vi "logTof.vi"(8 "ToF Reading":T1, 9 "Index":i32) -> ()   [LabVIEW 2014]
uses:
  Type Defs/tofReading.ctl
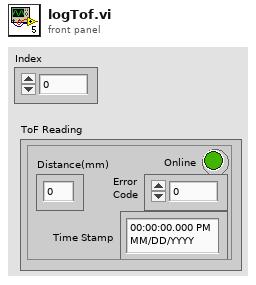
[diagram p1: front panel]
types:
  T1 = typedef "tofReading.ctl" = cluster{"Distance(mm)":u8, "Online":bool, "Error\nCode":u8, "Time Stamp":timestamp}
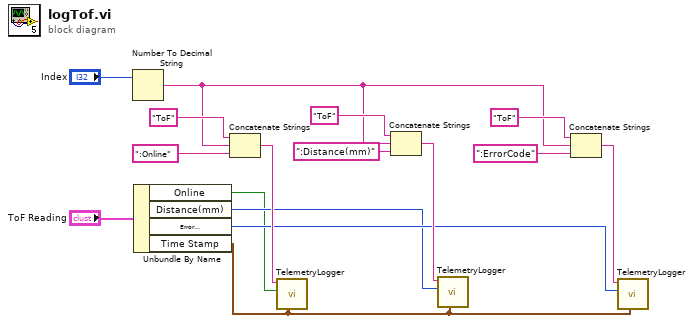
[diagram p0: block diagram]
diagram:
  n1 = Number To Decimal String(number="Index") -> (decimal integer string=w6:string)  [unwired: 1 in]
  n2 = Unbundle By Name("ToF Reading") -> ("Online"=w1:bool, "Distance(mm)"=w2:u8, "Error\nCode"=w3:u8, "Time Stamp"=w4:timestamp)
  n3 = Concatenate Strings("ToF", w6, ":Online") -> (w13:string)
  n4 = call "TelemetryLogger.vi"("Time Stamp"=w4, "Data"=w1, "Sensor:Reading"=w13) -> ()  [unwired: 9 in]
  n5 = Concatenate Strings("ToF", w6, ":Distance(mm)") -> (w12:string)
  n6 = call "TelemetryLogger.vi"("Time Stamp"=w4, "Data"=w2, "Sensor:Reading"=w12) -> ()  [unwired: 9 in]
  n7 = Concatenate Strings("ToF", w6, ":ErrorCode") -> (w7:string)
  n8 = call "TelemetryLogger.vi"("Time Stamp"=w4, "Data"=w3, "Sensor:Reading"=w7) -> ()  [unwired: 9 in]
